vi "read_T1_linux.vi"(11 "file_path":path) -> (0 "fitted_signal":T2, 1 "fit_parameters":T4 {"mse" format="%.3g"; "T1" format="%.3g"; "C1" format="%.3g"; "Tm" format="%.3g"; "Cm" format="%.3g"; "Ie" format="%.3g"}, 2 "T1_curve":T3, 3 "T1_parameters":T1, 4 "file_path":path, 5 "timetags":u32[][](array[numeric]), 7 "triggers":u32[][](array[numeric]))   [LabVIEW 2014]
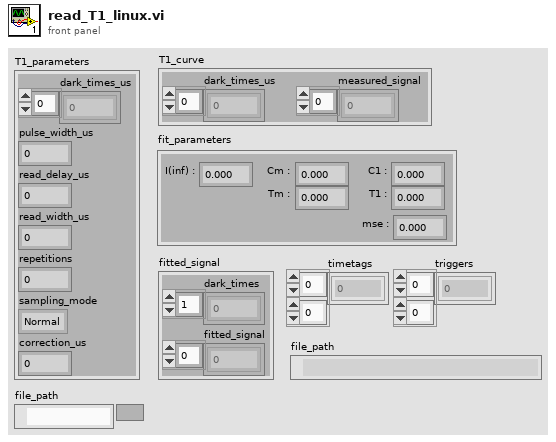
[diagram p1: front panel]
types:
  T1 = cluster{"dark_times_us":dbl[], "pulse_width_us":dbl, "read_delay_us":dbl, "read_width_us":dbl, "repetitions":i32, "sampling_mode":enum16{"Normal", "Sweep"}, "correction_us":dbl}
  T2 = cluster{"dark_times":dbl[], "fitted_signal":dbl[]}
  T3 = cluster{"dark_times_us":dbl[], "measured_signal":dbl[]}
  T4 = cluster{"Ie":dbl, "Cm":dbl, "Tm":dbl, "C1":dbl, "T1":dbl, "mse":dbl}
  T5 = enum16{"open", "replace", "create", "open or create", "replace or create", "replace or create with confirmation"}
  T6 = enum16{"Native", "Native Command Line", "UNIX", "Macintosh", "DOS"}
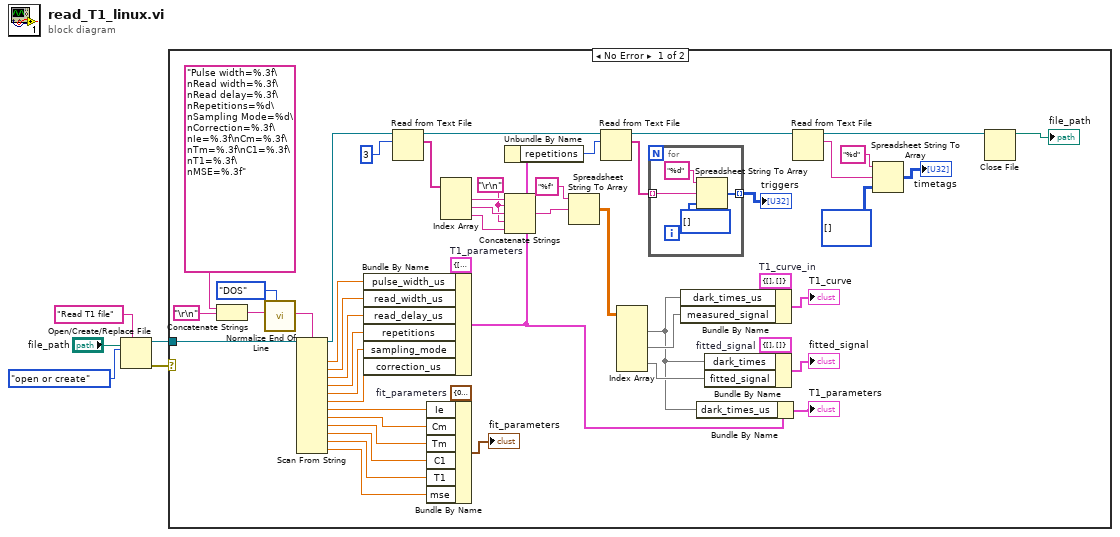
[diagram p0: block diagram]
diagram:
  n1 = Open/Create/Replace File(file path (use dialog)="file_path", prompt="Read T1 file", operation (0:open)=T5."open or create") -> (refnum out=w2:refnum<file>, error out=w3:errorcluster)  [unwired: 3 in, 1 out]
  n2 = case shown="No Error" w3 {
    tunnel: w2 -> [w20 _]
    frame No Error {
      w10 = "\r\n"
      w25 = T1 {"dark_times_us"=[], "pulse_width_us"=0.0, "read_delay_us"=0.0, "read_width_us"=0.0, "repetitions"=0, "sampling_mode"=enum."Normal", "correction_us"=0.0}  # T1_parameters
      w41 = T3 {"dark_times_us"=[], "measured_signal"=[]}  # T1_curve_in
      w42 = T2 {"dark_times"=[], "fitted_signal"=[]}  # fitted_signal
      w52 = T4 {"Ie"=0.0, "Cm"=0.0, "Tm"=0.0, "C1"=0.0, "T1"=0.0, "mse"=0.0}  # fit_parameters
      n3 = Concatenate Strings("Pulse width=%.3f\nRead width=%.3f\nRead delay=%.3f\nRepetitions=%d\nSampling Mode=%d\nCorrection=%.3f\nIe=%.3f\nCm=%.3f\nTm=%.3f\nC1=%.3f\nT1=%.3f\nMSE=%.3f" ("format string"), "\r\n") -> (w7:string)
      n4 = call <vilib>:"Normalize End Of Line.vi"("end of line (Native)"=T6."DOS", "string in"=w7) -> ("string out"=w11:string)  [unwired: 6 in]
      n5 = Scan From String(w11, w20) -> (w44:refnum<file>, output 1=w53:dbl, output 2=w54:dbl, output 3=w55:dbl, output 4=w56:dbl, output 5=w24:dbl, output 6=w23:dbl, output 7=w50:dbl, output 8=w49:dbl, output 9=w48:dbl, output 10=w47:dbl, output 11=w46:dbl, output 12=w45:dbl)  [unwired: 13 in, 1 out]
      n6 = Bundle By Name(cluster=w25, "pulse_width_us"=w53, "read_width_us"=w54, "read_delay_us"=w55, "repetitions"=w56, "sampling_mode"=w24, "correction_us"=w23) -> (w15:T1)
      n7 = Read from Text File(file (use dialog)=w44, count=3) -> (refnum out=w17:refnum<file>, text=w33:string[])  [unwired: 2 in, 2 out]
      n8 = Bundle By Name(cluster=w52, "Ie"=w50, "Cm"=w49, "Tm"=w48, "C1"=w47, "T1"=w46, "mse"=w45) -> (→"fit_parameters":T4)
      n9 = Index Array(array=w33) -> (element #1=w35:string, element #2=w27:string, element #3=w26:string)  [unwired: 3 in]
      n10 = Unbundle By Name(w15) -> ("repetitions"=w14:i32)
      n11 = Concatenate Strings(w35, w10, w27, w10, w26) -> (w32:string)
      n12 = Spreadsheet String To Array(format string="%f", spreadsheet string=w32) -> (array=w38:dbl[][])  [unwired: 2 in]
      n13 = Read from Text File(file (use dialog)=w17, count=w14) -> (refnum out=w16:refnum<file>, text=w13:string[])  [unwired: 2 in, 2 out]
      n14 = Index Array(array=w38) -> (element #1=w21:dbl[], element #2=w37:dbl[], element #3=w36:dbl[])  [unwired: 6 in]
      n15 = for {
        tunnel: w13 -> [w58] mode=indexing
        tunnel: [w57] -> w12 mode=indexing
        n16 = Spreadsheet String To Array(format string="%d", spreadsheet string=w58, array type (2D Dbl)=u32[] [] ("triggers")) -> (array=w57:u32[])  [unwired: 1 in]
      }
      "triggers" <- w12
      n17 = Bundle By Name(cluster=w41, "dark_times_us"=w21, "measured_signal"=w37) -> (→"T1_curve":T3)
      n18 = Bundle By Name(cluster=w15, "dark_times_us"=w21) -> (→"T1_parameters":T1)
      n19 = Bundle By Name(cluster=w42, "dark_times"=w21, "fitted_signal"=w36) -> (→"fitted_signal":T2)
      n20 = Read from Text File(file (use dialog)=w16) -> (refnum out=w19:refnum<file>, text=w30:string)  [unwired: 3 in, 2 out]
      n21 = Spreadsheet String To Array(format string="%d", spreadsheet string=w30, array type (2D Dbl)=u32[][] []) -> (array=→"timetags":u32[][])  [unwired: 1 in]
      n22 = Close File(refnum=w19) -> (path=→"file_path":path)  [unwired: 1 in, 1 out]
    }
    frame Error {
    }
  }
